vi "Descanner2_Analog_PMT_preGenFrame.vi"(0 "Pix":i32, 1 "scanPix":i32, 2 "delta_p":i32, 3 "Data":dbl[](array[numeric])) -> (5 "2Lines":dbl[][](array[numeric]))   [LabVIEW 2009]
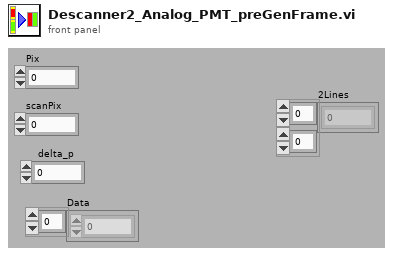
[diagram p1: front panel]
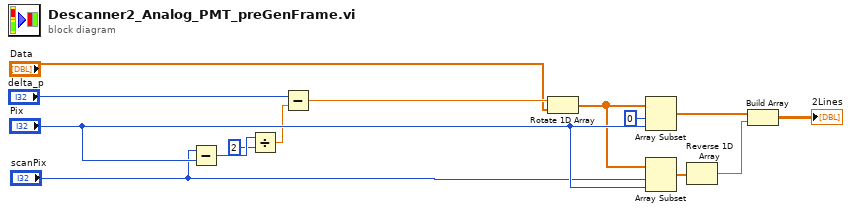
[diagram p0: block diagram]
diagram:
  n1 = Subtract(x="scanPix", y="Pix") -> (x-y=w14:i32)
  n2 = Divide(x=w14, y=2) -> (x/y=w4:dbl)
  n3 = Subtract(x="delta_p", y=w4) -> (x-y=w9:dbl)
  n4 = Rotate 1D Array(1:"Data", 2:w9) -> (0:w3:dbl[])
  n5 = Array Subset(array=w3, index=0, length="Pix") -> (w5:dbl[])
  n6 = Array Subset(array=w3, index="scanPix", length="Pix") -> (w10:dbl[])
  n7 = Reverse 1D Array(array=w10) -> (reversed array=w7:dbl[])
  n8 = Build Array(w5, w7) -> (→"2Lines":dbl[][])
